vi "DiscoverCommonTypeDefCallers.vi"(8 "Error In":errorcluster, 11 "Application Reference":refnum<vi>) -> (0 "Error Out":errorcluster, 2 "Dependendent TypeDefs wParents":T1(array[cluster]))   [LabVIEW 2013]
panel:
  out "loop iterations":i32
  out "All VIs containing moded TypeDefs":string[](array[string])
  out "All TypeDefs in memory":string[](array[string])
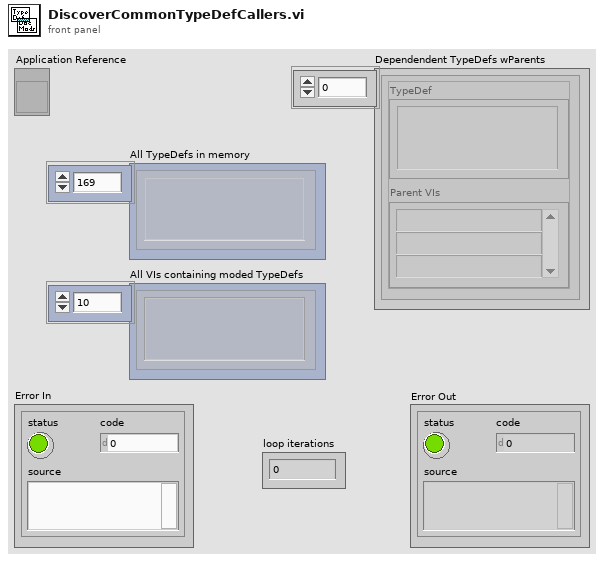
[diagram p1: front panel]
types:
  T1 = cluster{"TypeDef":string, "Parent VIs":string[]}[]
  T2 = cluster{"TypeDefName":string, "CtrlVIType":enum32{"not a control VI", "control", "typedef", "strict typedef"}}[]
  T3 = cluster{"ItemName":string, "VIType":enum32{"invalid VI type", "Standard VI", "Control VI", "Global VI", "Polymorphic VI", "Configuration VI", "SubSystem", "Facade VI", "Method VI", "Statechart Diagram VI"}, "Mods.Block Diagram":u32, "Mods.Front Panel":u32, "Mods.VI":u64}[]
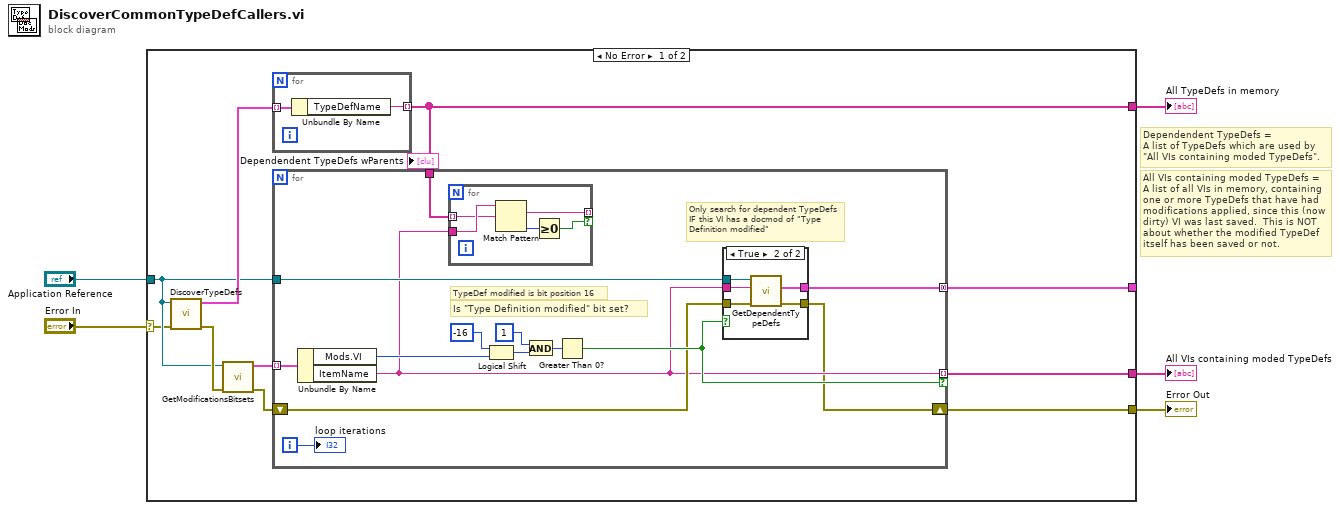
[diagram p0: block diagram]
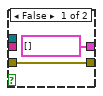
[diagram p2: hidden frame]
diagram:
  # "Dependendent TypeDefs =\nA list of TypeDefs which are used by \"All VIs containing moded TypeDefs\"."
  # "All VIs containing moded TypeDefs =\nA list of all VIs in memory, containing one or more TypeDefs that have had modifications applied, since this (now dirty) VI was last saved.  This is NOT about whether the modified TypeDef itself has been saved or not."
  n1 = case shown="No Error" "Error In" {
    selector: "Error In" -> [w6 w44]
    tunnel: [w15 w44] -> w5
    tunnel: [w14 _] -> w3
    tunnel: [w13 _] -> w4
    tunnel: [w12 _] -> _
    tunnel: "Application Reference" -> [w8 _]
    frame No Error {
      n2 = call "DiscoverTypeDefs.vi"("Error In"=w6, "Application Reference"=w8) -> ("Error Out"=w11:errorcluster, "All TypeDefs in Memory"=w10:T2)  [unwired: 7 in, 1 out]
      n3 = call "GetModificationsBitsets.vi"("Error In"=w11, "Application Reference"=w8) -> ("Error Out"=w7:errorcluster, "DocMods for All Items in Memory"=w9:T3)  [unwired: 8 in]
      n4 = for {
        tunnel: w10 -> [w17] mode=indexing
        tunnel: [w16] -> w13 mode=indexing
        n5 = Unbundle By Name(w17) -> ("TypeDefName"=w16:string)
      }
      n6 = for {
        tunnel: w9 -> [w31] mode=indexing
        shift-right: [w20] -> w15
        shift-left: w7 -> [w22]
        tunnel: [w21] -> w14 mode=indexing if=w24
        tunnel: w13 -> [w25]
        tunnel: w8 -> [w23]
        tunnel: [w18] -> w12 mode=concatenating
        i -> [w19]
        # "Only search for dependent TypeDefs IF this VI has a docmod of \"Type Definition modified\""
        # "TypeDef modified is bit position 16"
        # "Is \"Type Definition modified\" bit set?"
        n7 = Unbundle By Name(w31) -> ("Mods.VI"=w30:u64, "ItemName"=w21:string)
        n8 = for {
          tunnel: w21 -> [w43]
          tunnel: [w40] -> _ mode=indexing if=w39
          tunnel: w25 -> [w41] mode=indexing
          n9 = Match Pattern(string=w43, regular expression=w41) -> (match substring=w40:string, offset past match=w42:i32)  [unwired: 1 in, 2 out]
          n10 = Greater Or Equal To 0?(x=w42) -> (x >= 0?=w39:bool)
        }
        n11 = Logical Shift(y=i16 -16 ("x"), x=w30) -> (x << y=w28:u64)
        n12 = And(x=u64 1 ("y"), y=w28) -> (x .and. y?=w26:u64)
        n13 = Greater Than 0?(x=w26) -> (x > 0?=w24:bool)
        n14 = case shown="True" w24 {
          tunnel: w22 -> [w33 w38]
          tunnel: [w33 w37] -> w20
          tunnel: w23 -> [_ w36]
          tunnel: w21 -> [_ w35]
          tunnel: [T1 [] ("Dependendent TypeDefs wParents") w34] -> w18
          frame False {
          }
          frame True {
            n15 = call "GetDependentTypeDefs.vi"("error in (no error)"=w38, "vi name"=w35, "app reference in"=w36) -> ("error out"=w37:errorcluster, "Dependendent TypeDefs wParents"=w34:T1)  [unwired: 6 in, 1 out]
          }
        }
        "loop iterations" <- w19
      }
    }
    frame Error {
    }
  }
  "Error Out" <- w5
  "All TypeDefs in memory" <- w4
  "All VIs containing moded TypeDefs" <- w3
